vi "Update Plugin Status.vi"(8 "error in (no error)":errorcluster, 11 "CIF_UI in":refnum<class "CIF_UI.lvclass">) -> (0 "error out":errorcluster, 3 "CIF_UI out":refnum<class "CIF_UI.lvclass">)   [LabVIEW 2021, in "CIF_UI.lvclass"]
uses:
  CIF_UI.lvclass
  CIF_UI.lvclass/CIF_UI.ctl
  <vilib>/Utility/miscctls.llb/LVMapReplaceAction.ctl
  CIFPluginManager/CIFPluginManager/gRPC/CIF_Manager_client/RPC Messages/cif_plugincore_StatusData_State.ctl
  CIFPluginManager/CIFPluginManager/gRPC/CIF_Manager_Client_Wrapper/CIFManagerClientWrapper.lvlib
  CIFCore/Grpc/CIFCoreWrapper/CIFCoreWrapper.lvlib
  CIFPluginManager/CIFPluginManager/gRPC/CIF_Manager_client/CIF_Manager_client.lvlib
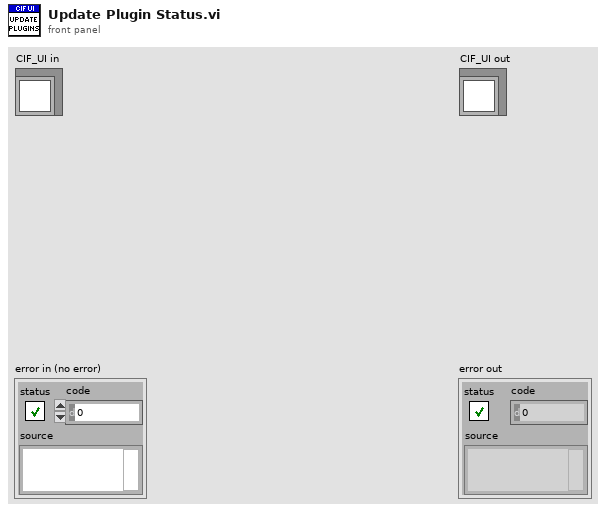
[diagram p1: front panel]
types:
  T1 = typedef "LVMapReplaceAction.ctl" = enum32{"Modify Entry only if found", "Add or Modify Entry", "Delete Entry"}
  T2 = typedef "CIF_Manager_client.lvlib/cif_plugincore_StatusData_State.ctl" = enum32{"NULL", "CREATING", "LISTENING", "RUNNING", "CLEANINGUP", "DESTROYING"}
  T3 = typedef "CIF_UI.lvclass/Plugin Connection Map.ctl" = map{string, T4}
  T4 = typedef "CIF_UI.lvclass/Plugin Connections.ctl" = cluster{"gRPC ID":T5, "Plugin info":T6}
  T5 = typedef "grpc-lvsupport-release.lvlib/grpcId.ctl" = u64
  T6 = typedef "CIF_Manager_client.lvlib/cif_manager_PluginInfo.ctl" = cluster{"plugin_name":string, "plugin_type":string, "grpc_port":i32, "plugin_version":T7, "status":T8}
  T7 = typedef "CIF_Manager_client.lvlib/cif_manager_PluginVersion.ctl" = cluster{"major_version":i32, "minor_version":i32, "fix_version":i32, "build_version":i32}
  T8 = typedef "CIF_Manager_client.lvlib/cif_plugincore_StatusData.ctl" = cluster{"state":T2, "timing_statistics":T9, "fifo_statistics":T11, "error":T12, "monitor_doubles":T13, "monitor_u64s":T14, "monitor_i64s":T15}
  T9 = typedef "CIF_Manager_client.lvlib/cif_plugincore_TimingStatistics.ctl" = cluster{"period":T10, "wake_error":T10, "execute":T10, "housekeep":T10, "idle":T10}
  T10 = typedef "CIF_Manager_client.lvlib/cif_plugincore_TimingStatsBasic.ctl" = cluster{"max":i32, "min":i32}
  T11 = typedef "CIF_Manager_client.lvlib/cif_plugincore_FifoStatistics.ctl" = cluster{"from_t0":T10, "from_previous_plugin":T10, "output_error":T10}
  T12 = typedef "CIF_Manager_client.lvlib/cif_plugincore_Error.ctl" = cluster{"status":bool, "code":i32}
  T13 = typedef "CIF_Manager_client.lvlib/cif_plugincore_MonitorDoubles.ctl" = cluster{"double_1":dbl, "double_2":dbl, "double_3":dbl, "double_4":dbl}
  T14 = typedef "CIF_Manager_client.lvlib/cif_plugincore_MonitorU64.ctl" = cluster{"u64_1":u64, "u64_2":u64, "u64_3":u64, "u64_4":u64}
  T15 = typedef "CIF_Manager_client.lvlib/cif_plugincore_MonitorI64.ctl" = cluster{"i64_1":i64, "i64_2":i64, "i64_3":i64, "i64_4":i64}
  T16 = typedef "CIFCoreCommon.lvlib/gRPC Reported Plugin Status.ctl" = cluster{"State":T17, "Timing Statistics (us)":T18, "FIFO Statistics (us)":T20, "error":T21, "Monitor Doubles":T22, "Monitor U64":T23, "Monitor I64":T24}
  T17 = typedef "CIFCoreCommon.lvlib/Plugin State.ctl" = enum32{"Null", "Creating", "Listening", "Running", "CleaningUp", "Destroying"}
  T18 = typedef "CIFCoreCommon.lvlib/Timing Statistics.ctl" = cluster{"Period":T19, "Wake Error":T19, "Execute":T19, "Housekeep":T19, "Idle":T19}
  T19 = typedef "CIFCoreCommon.lvlib/Timing Stats Base.ctl" = cluster{"Max":i32, "Min":i32}
  T20 = typedef "CIFCoreCommon.lvlib/FIFO Statistics.ctl" = cluster{"From T0":T19, "From Previous Plugin":T19, "Output Error":T19}
  T21 = typedef "CIFCoreCommon.lvlib/Simple Error.ctl" = cluster{"status":bool, "code":i32}
  T22 = typedef "CIFCoreCommon.lvlib/Monitor Doubles.ctl" = cluster{"1":dbl, "2":dbl, "3":dbl, "4":dbl}
  T23 = typedef "CIFCoreCommon.lvlib/Monitor U64.ctl" = cluster{"1":u64, "2":u64, "3":u64, "4":u64}
  T24 = typedef "CIFCoreCommon.lvlib/Monitor I64.ctl" = cluster{"1":i64, "2":i64, "3":i64, "4":i64}
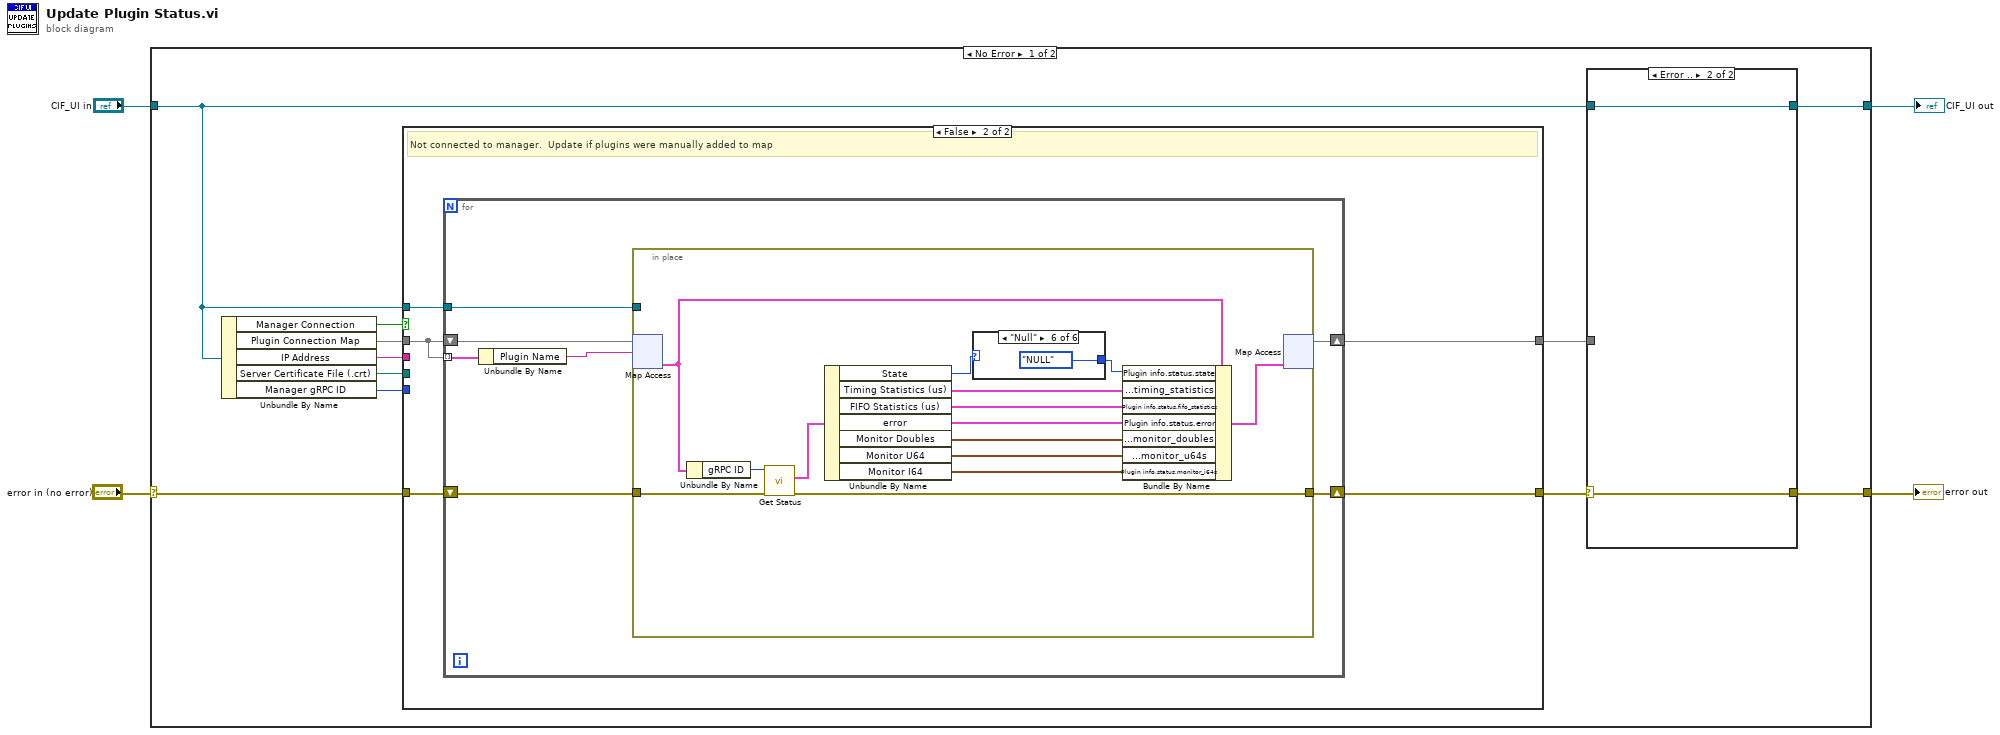
[diagram p0: block diagram]
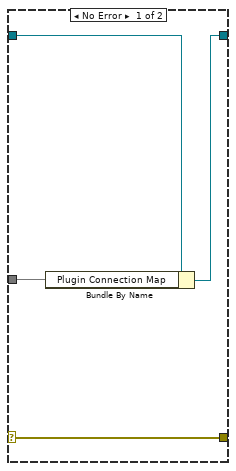
[diagram p2: hidden frame]
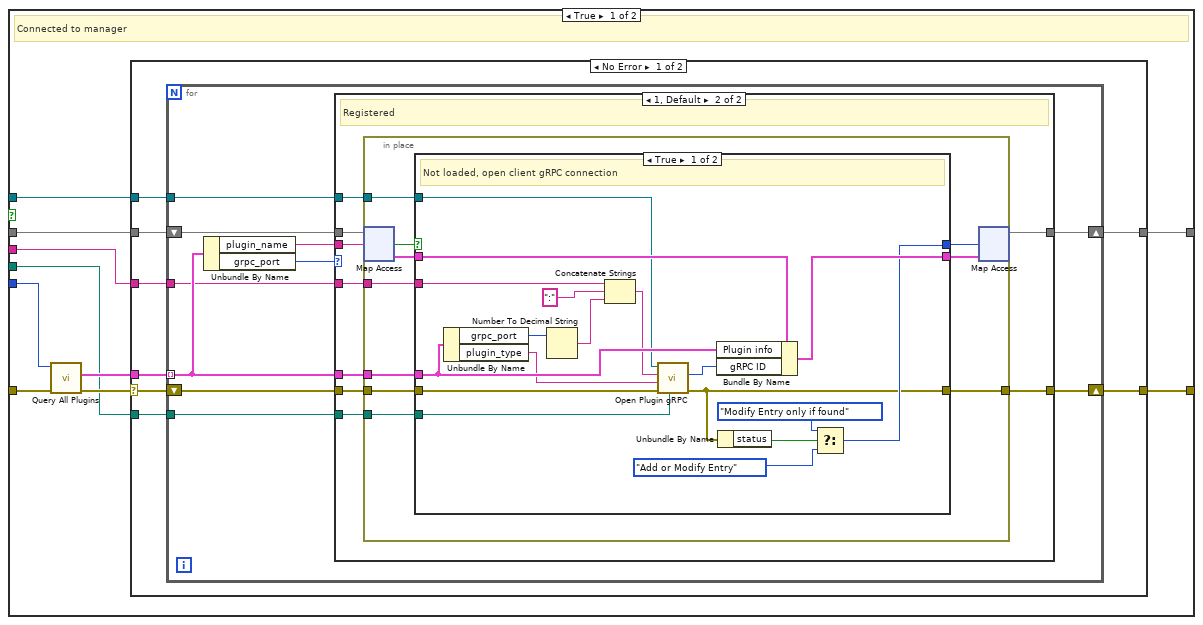
[diagram p3: hidden frame]
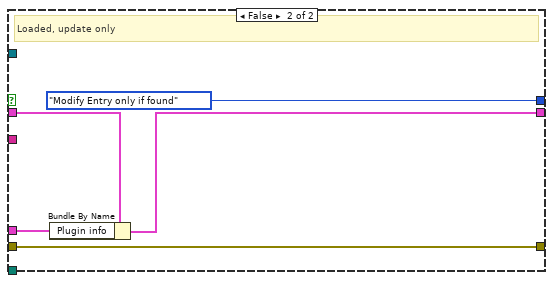
[diagram p5: hidden frame]
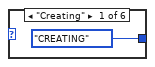
[diagram p7: hidden frame]
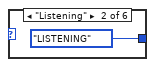
[diagram p8: hidden frame]
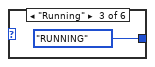
[diagram p9: hidden frame]
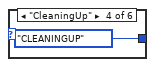
[diagram p10: hidden frame]
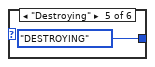
[diagram p11: hidden frame]
diagram:
  n1 = case shown="No Error" "error in (no error)" {
    selector: "error in (no error)" -> [w11 w129]
    tunnel: [w6 w129] -> w3
    tunnel: [w7 w128] -> w1
    tunnel: "CIF_UI in" -> [w9 w128]
    frame No Error {
      n2 = Unbundle By Name(w9) -> ("Manager Connection"=w10:bool, "Plugin Connection Map"=w15:T3, "IP Address"=w14:string, "Server Certificate File (.crt)"=w13:path, "Manager gRPC ID"=w12:T5)
      n3 = case shown="False" w10 {
        tunnel: w15 -> [w29 w96]
        tunnel: w14 -> [w28 _]
        tunnel: w13 -> [w27 _]
        tunnel: w12 -> [w26 _]
        tunnel: w11 -> [w25 w97]
        tunnel: [w22 w98] -> w5
        tunnel: w9 -> [w24 w100]
        tunnel: [w23 w99] -> w8
        frame True {
          # "Connected to manager"
          n4 = call "Query All Plugins.vi"("error in"=w25, "gRPC ID in"=w26) -> ("error out"=w31:errorcluster, "plugin_info"=w30:T6[])  [unwired: 7 in, 1 out]
          n5 = case shown="No Error" w31 {
            selector: w31 -> [w35 w95]
            tunnel: w30 -> [w39 _]
            tunnel: w29 -> [w38 w94]
            tunnel: w28 -> [w37 _]
            tunnel: w27 -> [w36 _]
            tunnel: [w34 w95] -> w22
            tunnel: [w33 w94] -> w23
            tunnel: w24 -> [w32 _]
            frame No Error {
              n6 = for {
                tunnel: w39 -> [w47] mode=indexing
                tunnel: w37 -> [w46]
                tunnel: w36 -> [w45]
                shift-right: [w42] -> w34
                shift-left: w35 -> [w44]
                shift-right: [w41] -> w33
                shift-left: w38 -> [w49]
                tunnel: w32 -> [w40]
                n7 = Unbundle By Name(w47) -> ("plugin_name"=w48:string, "grpc_port"=w43:i32)
                n8 = case shown="1, Default" w43 {
                  tunnel: w49 -> [w51 w60]
                  tunnel: w48 -> [_ w59]
                  tunnel: w47 -> [_ w58]
                  tunnel: w46 -> [_ w57]
                  tunnel: w45 -> [_ w56]
                  tunnel: w44 -> [w50 w55]
                  tunnel: [w50 w54] -> w42
                  tunnel: [w51 w53] -> w41
                  tunnel: w40 -> [_ w52]
                  frame -1, 0 {
                    # "Not a valid port.  Not yet registered"
                  }
                  frame 1, Default {
                    # "Registered"
                    n9 = in-place {
                      in-place-border: w58 -> [w69]
                      in-place-border: w57 -> [w67]
                      in-place-border: w56 -> [w66]
                      in-place-border: w55 -> [w65]
                      in-place-border: [w62] -> w54
                      in-place-border: w52 -> [w61]
                      n10 = in-place-map #1(w60, w59) -> (w68:T4, w70:bool)  [unwired: 1 in]
                      n11 = case shown="True" w70 {
                        tunnel: w69 -> [w85 w92]
                        tunnel: w68 -> [w86 w93]
                        tunnel: w67 -> [w79 _]
                        tunnel: w66 -> [w77 _]
                        tunnel: w65 -> [w76 w89]
                        tunnel: [w84 w91] -> w64
                        tunnel: [w80 LVMapReplaceAction."Modify Entry only if found" ("action")] -> w63
                        tunnel: [w75 w89] -> w62
                        tunnel: w61 -> [w73 _]
                        frame True {
                          # "Not loaded, open client gRPC connection"
                          n12 = Unbundle By Name(w85) -> ("grpc_port"=w88:i32, "plugin_type"=w71:string)
                          n13 = Number To Decimal String(number=w88) -> (decimal integer string=w87:string)  [unwired: 1 in]
                          n14 = Concatenate Strings(w79, ":" ("regular expression"), w87) -> (w72:string)
                          n15 = call-dynamic "Open Plugin gRPC.vi"("Server Certificate File (.crt)"=w77, "error in (no error)"=w76, "Type"=w71, "address"=w72, "CIF_UI in"=w73) -> ("error out"=w75:errorcluster, "gRPC ID Out"=w74:T5)  [unwired: 4 in, 1 out]
                          n16 = Bundle By Name(cluster=w86, "Plugin info"=w85, "gRPC ID"=w74) -> (w84:T4)
                          n17 = Unbundle By Name(w75) -> ("status"=w83:bool)
                          n18 = Select(t=LVMapReplaceAction."Modify Entry only if found", s=w83, f=LVMapReplaceAction."Add or Modify Entry" ("action")) -> (s? t:f=w80:T1)
                        }
                        frame False {
                          # "Loaded, update only"
                          n19 = Bundle By Name(cluster=w93, "Plugin info"=w92) -> (w91:T4)
                        }
                      }
                      n20 = in-place-map #1(w64, w63) -> (w53:T3)  [unwired: 2 out]
                    }
                  }
                }
              }
            }
            frame Error {
            }
          }
        }
        frame False {
          # "Not connected to manager.  Update if plugins were manually added to map"
          n21 = for {
            shift-right: [w105] -> w98
            shift-left: w97 -> [w106]
            shift-right: [w104] -> w99
            shift-left: w96 -> [w107]
            tunnel: w100 -> [w103]
            tunnel: w96 -> [w102] mode=indexing
            n22 = Unbundle By Name(w102) -> ("Plugin Name"=w101:string)
            n23 = in-place {
              in-place-border: w106 -> [w112]
              in-place-border: [w111] -> w105
              in-place-border: w103 -> [_]
              n24 = in-place-map #2(w107, w101) -> (w121:T4)  [unwired: 1 in, 1 out]
              n25 = Unbundle By Name(w121) -> ("gRPC ID"=w120:T5)
              n26 = call "Get Status.vi"("error in"=w112, "gRPC ID"=w120) -> ("error out"=w111:errorcluster, "Node Status"=w119:T16)  [unwired: 7 in, 1 out]
              n27 = Unbundle By Name(w119) -> ("State"=w108:T17, "Timing Statistics (us)"=w113:T18, "FIFO Statistics (us)"=w114:T20, "error"=w115:T21, "Monitor Doubles"=w116:T22, "Monitor U64"=w117:T23, "Monitor I64"=w118:T24)
              n28 = case shown="\"Null\"" w108 {
                tunnel: [cif_plugincore_StatusData_State."CREATING" ("Plugin info.status.state") cif_plugincore_StatusData_State."LISTENING" ("Plugin info.status.state") cif_plugincore_StatusData_State."RUNNING" ("Plugin info.status.state") cif_plugincore_StatusData_State."CLEANINGUP" ("Plugin info.status.state") cif_plugincore_StatusData_State."DESTROYING" ("Plugin info.status.state") cif_plugincore_StatusData_State."NULL" ("Plugin info.status.state")] -> w109
                frame "Creating" {
                }
                frame "Listening" {
                }
                frame "Running" {
                }
                frame "CleaningUp" {
                }
                frame "Destroying" {
                }
                frame "Null" {
                }
              }
              n29 = Bundle By Name(cluster=w121, "Plugin info.status.state"=w109, "Plugin info.status.timing_statistics"=w113, "Plugin info.status.fifo_statistics"=w114, "Plugin info.status.error"=w115, "Plugin info.status.monitor_doubles"=w116, "Plugin info.status.monitor_u64s"=w117, "Plugin info.status.monitor_i64s"=w118) -> (w110:T4)
              n30 = in-place-map #2(w110) -> (w104:T3)  [unwired: 1 in, 2 out]
            }
          }
        }
      }
      n31 = case shown="Error .." w5 {
        selector: w5 -> [w16 w20]
        tunnel: w8 -> [w19 _]
        tunnel: w9 -> [w18 w21]
        tunnel: [w17 w21] -> w7
        tunnel: [w16 w20] -> w6
        frame No Error {
          n32 = Bundle By Name(cluster=w18, "Plugin Connection Map"=w19) -> (w17:refnum<class "CIF_UI.lvclass">)
        }
        frame Error {
        }
      }
    }
    frame Error {
    }
  }
  "error out" <- w3
  "CIF_UI out" <- w1
